vi "제목없음 2.vi"   [LabVIEW 2014]
uses:
  <vilib>/Utility/sysdir.llb/System Directory Type.ctl
types:
  T1 = typedef "System Directory Type.ctl" = i32
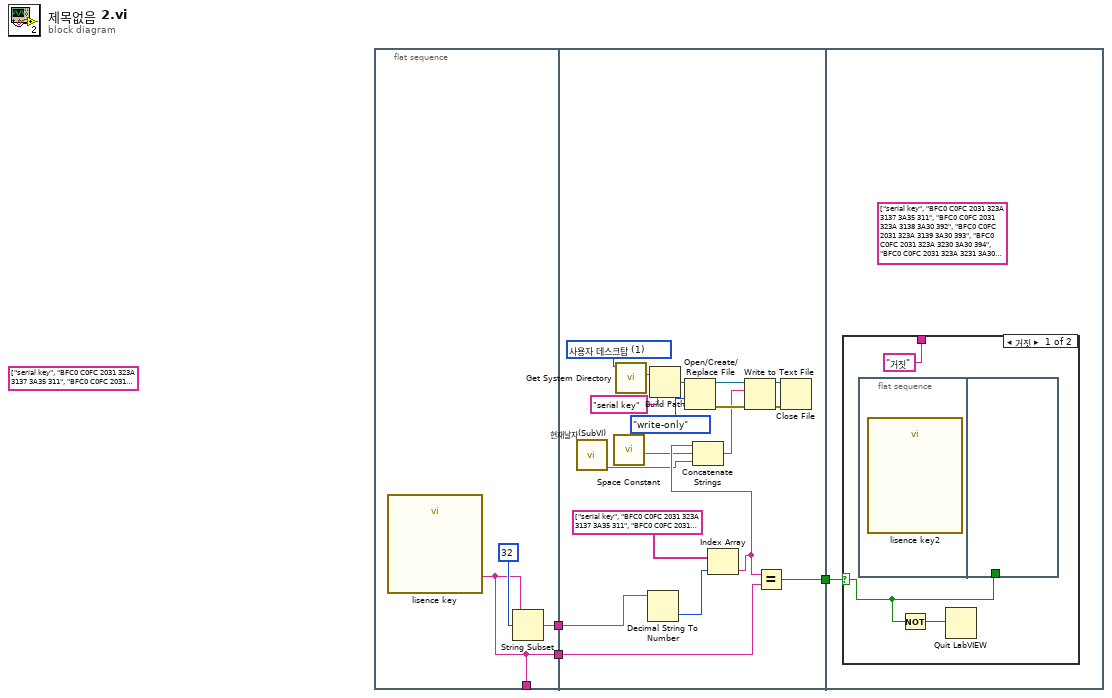
[diagram p0: block diagram]
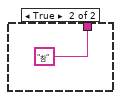
[diagram p2: hidden frame]
diagram:
  (unwired) string[] ["serial key", "BFC0 C0FC 2031 323A 3137 3A35 311", "BFC0 C0FC 2031 323A 3138 3A30 392", "BFC0 C0FC 2031 323A 3139 3A30 393", "BFC0 C0FC 2031 323A 3230 3A30 394", "BFC0 C0FC 2031 323A 3231 3A30 395", "BFC0 C0FC 2031 323A 3232 3A30 396", "BFC0 C0FC 2031 323A 3233 3A30 397", "BFC0 C0FC 2031 323A 3234 3A30 398", "BFC0 C0FC 2031 323A 3235 3A30 399", "BFC0 C0FC 2031 323A 3236 3A30 3910", "BFC0 C0FC 2031 323A 3237 3A30 3911", "BFC0 C0FC 2031 323A 3238 3A30 3912", "BFC0 C0FC 2031 323A 3239 3A30 3913", "BFC0 C0FC 2031 323A 3036 3A33 3214", "BFC0 C0FC 2031 323A 3037 3A33 3215", "BFC0 C0FC 2031 323A 3038 3A33 3216", "BFC0 C0FC 2031 323A 3038 3A33 3217", "BFC0 C0FC 2031 323A 3039 3A33 3218", "BFC0 C0FC 2031 323A 3039 3A35 3019", "BFC0 C0FC 2031 323A 3130 3A35 3020", "BFC0 C0FC 2031 323A 3131 3A35 3121", "BFC0 C8C4 2031 313A 3536 3A33 3222", "BFC0 C8C4 2031 313A 3537 3A33 3223", "BFC0 C8C4 2031 313A 3538 3A33 3224", "BFC0 C8C4 2031 313A 3539 3A33 3225", "BFC0 C0FC 2031 323A 3030 3A33 3226", "BFC0 C0FC 2031 323A 3031 3A33 3227", "BFC0 C0FC 2031 323A 3032 3A33 3228", "BFC0 C0FC 2031 323A 3033 3A33 3229", "BFC0 C0FC 2031 323A 3034 3A33 3230", "BFC0 C0FC 2031 323A 3035 3A33 3231", "BFC0 C0FC 2031 323A 3036 3A33 3232", "BFC0 C0FC 2031 323A 3037 3A33 3233", "BFC0 C0FC 2031 323A 3038 3A33 3234", ""] ("출력 배열")
  n1 = flat-sequence {
    tunnel: [w5] -> w3
    tunnel: [w4] -> w2
    tunnel: [w4] -> _
    tunnel: w3 -> [w24]
    tunnel: [w7] -> w1
    tunnel: w2 -> [w22]
    tunnel: w1 -> [w25]
    frame #0 {
      n2 = call "lisence key"() -> ("lisence key"=w4:string)  [unwired: 17 in, 2 out]
      n3 = String Subset(string=w4, offset (0)=32 ("오프셋(0)")) -> (substring=w5:string)  [unwired: 1 in]
    }
    frame #1 {
      w15 = T1 1 items=["사용자 홈"=0, "사용자 데스크탑"=1, "사용자 문서"=2, "사용자 어플리케이션 데이터"=3, "사용자 환경"=4, "사용자 임시"=5, "퍼블릭 문서"=6, "퍼블릭 어플리케이션 데이터"=7, "퍼블릭 환경"=8, "퍼블릭 캐시"=13, "시스템 코어 라이브러리"=9, "시스템 설치된 라이브러리"=10, "어플리케이션 파일"=11, "부팅 볼륨 루트"=12] ("system directory type")
      n4 = call "현재날자(SubVI).vi"() -> ("월,일 을 문자열로"=w9:string)  [unwired: 5 in, 6 out]
      n5 = call <vilib>:"Space Constant.vi"() -> ("String"=w8:string)
      n6 = call <vilib>:"Get System Directory.vi"("system directory type"=w15) -> ("system directory"=w14:path)  [unwired: 10 in]
      n7 = Decimal String To Number(string=w24) -> (number=w23:i32)  [unwired: 2 in, 1 out]
      n8 = Build Path(base path=w14, name or relative path="serial key" ("이름 또는 상대 경로")) -> (appended path=w13:path)
      n9 = Open/Create/Replace File(file path (use dialog)=w13, access (0:read/write)=enum16{"read/write", "read-only", "write-only"}."write-only" ("접근(0:읽기/쓰기)")) -> (refnum out=w21:refnum<file>, error out=w20:errorcluster)  [unwired: 4 in, 1 out]
      n10 = Index Array(array=string[] ["serial key", "BFC0 C0FC 2031 323A 3137 3A35 311", "BFC0 C0FC 2031 323A 3138 3A30 392", "BFC0 C0FC 2031 323A 3139 3A30 393", "BFC0 C0FC 2031 323A 3230 3A30 394", "BFC0 C0FC 2031 323A 3231 3A30 395", "BFC0 C0FC 2031 323A 3232 3A30 396", "BFC0 C0FC 2031 323A 3233 3A30 397", "BFC0 C0FC 2031 323A 3234 3A30 398", "BFC0 C0FC 2031 323A 3235 3A30 399", "BFC0 C0FC 2031 323A 3236 3A30 3910", "BFC0 C0FC 2031 323A 3237 3A30 3911", "BFC0 C0FC 2031 323A 3238 3A30 3912", "BFC0 C0FC 2031 323A 3239 3A30 3913", "BFC0 C0FC 2031 323A 3036 3A33 3214", "BFC0 C0FC 2031 323A 3037 3A33 3215", "BFC0 C0FC 2031 323A 3038 3A33 3216", "BFC0 C0FC 2031 323A 3038 3A33 3217", "BFC0 C0FC 2031 323A 3039 3A33 3218", "BFC0 C0FC 2031 323A 3039 3A35 3019", "BFC0 C0FC 2031 323A 3130 3A35 3020", "BFC0 C0FC 2031 323A 3131 3A35 3121", "BFC0 C8C4 2031 313A 3536 3A33 3222", "BFC0 C8C4 2031 313A 3537 3A33 3223", "BFC0 C8C4 2031 313A 3538 3A33 3224", "BFC0 C8C4 2031 313A 3539 3A33 3225", "BFC0 C0FC 2031 323A 3030 3A33 3226", "BFC0 C0FC 2031 323A 3031 3A33 3227", "BFC0 C0FC 2031 323A 3032 3A33 3228", "BFC0 C0FC 2031 323A 3033 3A33 3229", "BFC0 C0FC 2031 323A 3034 3A33 3230", "BFC0 C0FC 2031 323A 3035 3A33 3231", "BFC0 C0FC 2031 323A 3036 3A33 3232", "BFC0 C0FC 2031 323A 3037 3A33 3233", "BFC0 C0FC 2031 323A 3038 3A33 3234", ""] ("출력 배열"), index=w23) -> (element=w10:string)
      n11 = Concatenate Strings(w10, w8, w9) -> (w12:string)
      n12 = Write to Text File(file (use dialog)=w21, text=w12, error in=w20) -> (refnum out=w18:refnum<file>, error out=w19:errorcluster)  [unwired: 1 in, 1 out]
      n13 = Equal?(x=w10, y=w22) -> (x = y?=w7:bool)
      n14 = Close File(refnum=w18, error in=w19) -> ()  [unwired: 2 out]
    }
    frame #2 {
      (unwired) string[] ["serial key", "BFC0 C0FC 2031 323A 3137 3A35 311", "BFC0 C0FC 2031 323A 3138 3A30 392", "BFC0 C0FC 2031 323A 3139 3A30 393", "BFC0 C0FC 2031 323A 3230 3A30 394", "BFC0 C0FC 2031 323A 3231 3A30 395", "BFC0 C0FC 2031 323A 3232 3A30 396", "BFC0 C0FC 2031 323A 3233 3A30 397", "BFC0 C0FC 2031 323A 3234 3A30 398", "BFC0 C0FC 2031 323A 3235 3A30 399", "BFC0 C0FC 2031 323A 3236 3A30 3910", "BFC0 C0FC 2031 323A 3237 3A30 3911", "BFC0 C0FC 2031 323A 3238 3A30 3912", "BFC0 C0FC 2031 323A 3239 3A30 3913", "BFC0 C0FC 2031 323A 3036 3A33 3214", "BFC0 C0FC 2031 323A 3037 3A33 3215", "BFC0 C0FC 2031 323A 3038 3A33 3216", "BFC0 C0FC 2031 323A 3038 3A33 3217", "BFC0 C0FC 2031 323A 3039 3A33 3218", "BFC0 C0FC 2031 323A 3039 3A35 3019", "BFC0 C0FC 2031 323A 3130 3A35 3020", "BFC0 C0FC 2031 323A 3131 3A35 3121", "BFC0 C8C4 2031 313A 3536 3A33 3222", "BFC0 C8C4 2031 313A 3537 3A33 3223", "BFC0 C8C4 2031 313A 3538 3A33 3224", "BFC0 C8C4 2031 313A 3539 3A33 3225", "BFC0 C0FC 2031 323A 3030 3A33 3226", "BFC0 C0FC 2031 323A 3031 3A33 3227", "BFC0 C0FC 2031 323A 3032 3A33 3228", "BFC0 C0FC 2031 323A 3033 3A33 3229", "BFC0 C0FC 2031 323A 3034 3A33 3230", "BFC0 C0FC 2031 323A 3035 3A33 3231", "BFC0 C0FC 2031 323A 3036 3A33 3232", "BFC0 C0FC 2031 323A 3037 3A33 3233", "BFC0 C0FC 2031 323A 3038 3A33 3234", ""] ("출력 배열")
      n15 = case shown="거짓" w25 {
        selector: w25 -> [w27 _]
        tunnel: ["거짓" "참"] -> _
        frame False {
          n16 = flat-sequence {
            tunnel: w27 -> [_]
            frame #0 {
              n17 = call "lisence key2"() -> ()  [unwired: 10 in, 2 out]
            }
            frame #1 {
            }
          }
          n18 = Not(x=w27) -> (.not. x?=w26:bool)
          n19 = Quit LabVIEW(quit? (T)=w26) -> ()
        }
        frame True {
        }
      }
    }
  }
